vi "Align tilt stages.vi"() -> ()   [LabVIEW 2013]
uses:
  <vilib>/Utility/file.llb/Read From Spreadsheet File (I64).vi
  <vilib>/Utility/file.llb/Write To Spreadsheet File (I64).vi
  <instrlib>/ZaberTSeries/ZaberTSeries.lvlib
panel:
  in  "Load saved position":bool=TRUE
  in  "Save position":bool=TRUE
  in  "Path for saved position":path=path "C:/Users/lab/Documents/GitHub/single-photon-vision/Tools/Calibration/position.txt"
  out "Current position (RV)":i32
  out "Current position (RH)":i32
  in  "Device Number (RH)":u8=4
  in  "Device Number (RV)":u8=3
  out "Current position (LH)":i32
  in  "Device Number (LH)":u8=1
  out "Current position (LV)":i32
  out "error out":errorcluster
  in  "Step Size":i32=1000
  in  "Device Number (LV)":u8=2
  in  "error in (no error)":errorcluster
  in  "VISA resource name":refnum<visa-resource-name>="COM5"
  in  "stop":bool
  # "Press space to update from saved positions."
  # "Press space after STOP to end the VI."
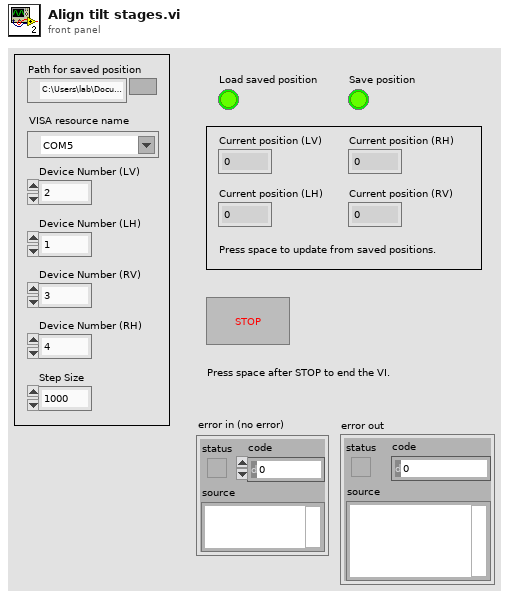
[diagram p1: front panel]
types:
  T1 = enum16{"0", "1", "2", "3", "4", "5", "6", "7", "8", "9", "A", "B", "C", "D", "E", "F", "G", "H", "I", "J", "K", "L", "M", "N", "O", "P", "Q", "R", "S", "T", "U", "V", "W", "X", "Y", "Z", "F1", "F2", "F3", "F4", "F5", "F6", "F7", "F8", "F9", "F10", "F11", "F12", "F13", "F14", "F15", "ADD", "BACK", "BACKSLASH", "CAPITAL", "COMMA", "DECIMAL", "DELETE", "DIVIDE", "DOWN", "END", "EQUALS", "ESCAPE", "GRAVE (`)", "HOME", "INSERT", "LBRACKET", "LCONTROL", "LEFT", "L ALT", "LSHIFT", "LWIN", "MINUS", "MULTIPLY", "NEXT", "NUMLOCK", "NUMPAD_0", "NUMPAD_1", "NUMPAD_2", "NUMPAD_3", "NUMPAD_4", "NUMPAD_5", "NUMPAD_6", "NUMPAD_7", "NUMPAD_8", "NUMPAD_9", "PAUSE", "PERIOD", "PRIOR (PG UP)", "RBRACKET", "RCONTROL", "RETURN", "RIGHT", "R ALT", "RSHIFT", "RWIN", "SCROLL", "SEMICOLON", "SLASH", "SPACE", "SUBTRACT", "TAB", "UP", "ENTER (num pad)", "' (quote)"}
  T2 = cluster{"Response Count":i32, "Command":u8, "Response Count":i32, "Response Count":i32}
  T3 = typedef "ZaberTSeries.lvlib/Response.ctl" = cluster{"Device Number":u8, "Command":u8, "Data":i32}
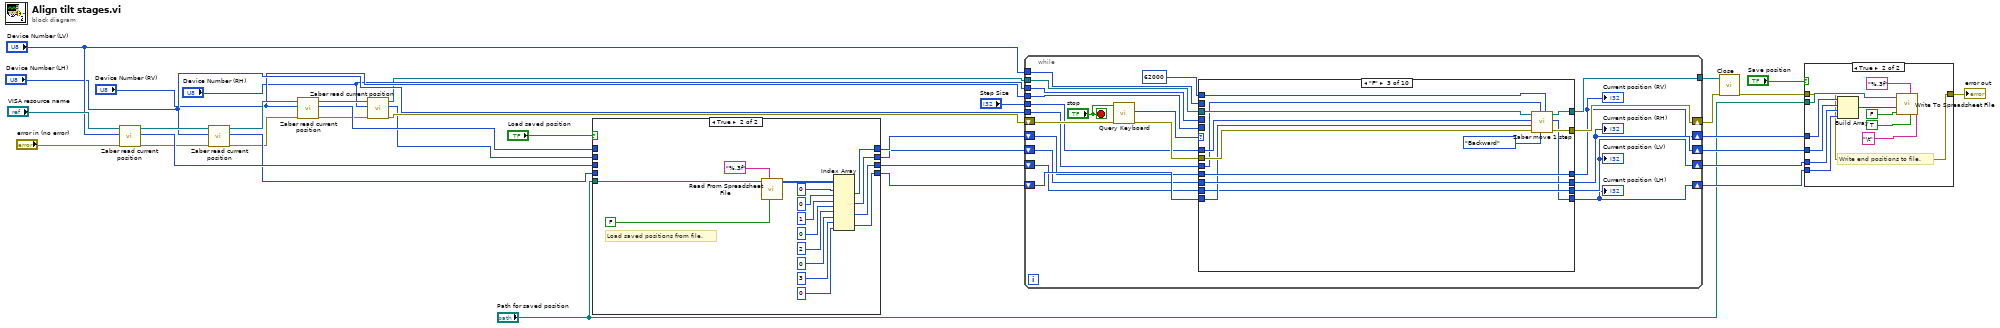
[diagram p0: block diagram]
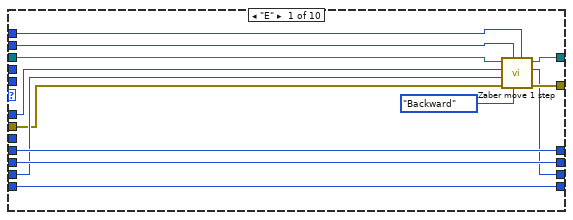
[diagram p4: hidden frame]
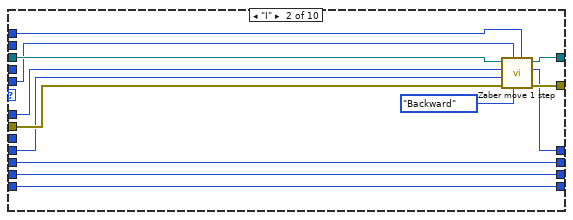
[diagram p5: hidden frame]
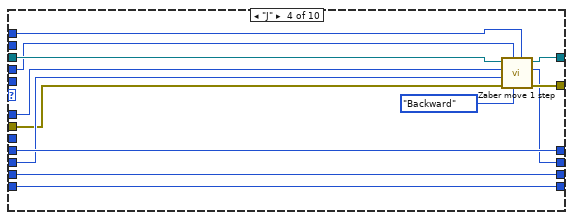
[diagram p6: hidden frame]
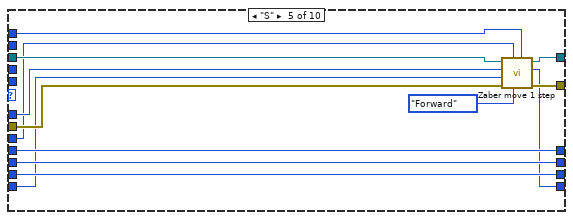
[diagram p7: hidden frame]
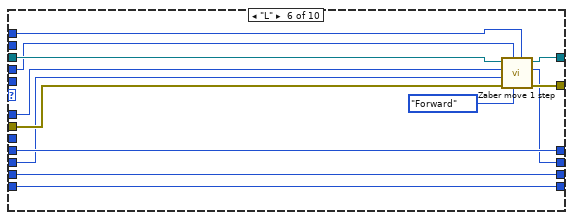
[diagram p8: hidden frame]
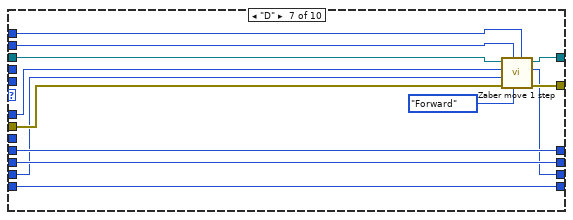
[diagram p9: hidden frame]
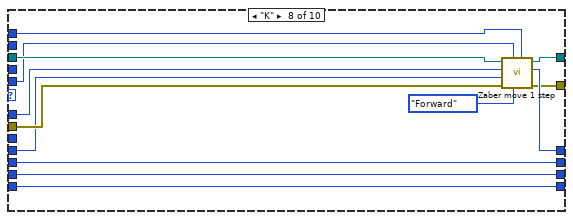
[diagram p10: hidden frame]
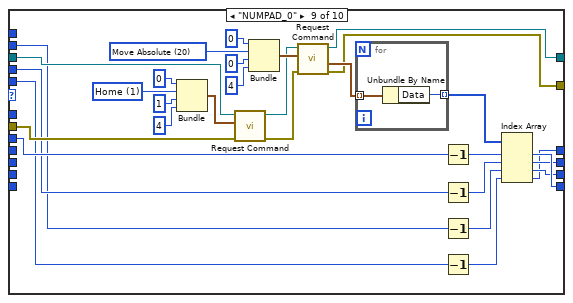
[diagram p11: hidden frame]
diagram:
  n1 = call "Zaber read current position.vi"("error in (no error)"="error in (no error)", "Device Number (LV)"="Device Number (LV)", "VISA Refnum in"="VISA resource name") -> ("error out"=w14:errorcluster, "Current position (LV)"=w18:i32, "VISA Refnum out"=w13:refnum<visa-resource-name>)  [unwired: 6 in]
  n2 = call "Zaber read current position.vi"("error in (no error)"=w14, "Device Number (LV)"="Device Number (LH)", "VISA Refnum in"=w13) -> ("error out"=w10:errorcluster, "Current position (LV)"=w11:i32, "VISA Refnum out"=w9:refnum<visa-resource-name>)  [unwired: 6 in]
  n3 = call "Zaber read current position.vi"("error in (no error)"=w10, "Device Number (LV)"="Device Number (RV)", "VISA Refnum in"=w9) -> ("error out"=w6:errorcluster, "Current position (LV)"=w7:i32, "VISA Refnum out"=w5:refnum<visa-resource-name>)  [unwired: 6 in]
  n4 = call "Zaber read current position.vi"("error in (no error)"=w6, "Device Number (LV)"="Device Number (RH)", "VISA Refnum in"=w5) -> ("error out"=w3:errorcluster, "Current position (LV)"=w2:i32, "VISA Refnum out"=w1:refnum<visa-resource-name>)  [unwired: 6 in]
  n5 = case shown="True" "Load saved position" {
    tunnel: "Path for saved position" -> [_ w54]
    tunnel: w7 -> [w38 _]
    tunnel: [w38 w43] -> w19
    tunnel: w18 -> [w37 _]
    tunnel: [w37 w41] -> w17
    tunnel: [w36 w40] -> w16
    tunnel: w11 -> [w36 _]
    tunnel: [w35 w42] -> w15
    tunnel: w2 -> [w35 _]
    frame False {
    }
    frame True {
      # "Load saved positions from file."
      n6 = call-poly <vilib>:"Read From Spreadsheet File.vi"("transpose (no:F)"=FALSE, "format (%d)"="%.3f" ("format (%.3f)"), "file path (dialog if empty)"=w54) -> ("all rows"=w39:i64[][])  [unwired: 4 in, 4 out]
      n7 = Index Array(array=w39, index (row) #1=0 ("index"), index (col) #1=0 ("disabled index (col)"), index (row) #2=1 ("index"), index (col) #2=0 ("disabled index (col)"), index (row) #3=2 ("index"), index (col) #3=0 ("disabled index (col)"), index (row) #4=3 ("index"), index (col) #4=0 ("disabled index (col)")) -> (element #1=w43:i64, element #2=w42:i64, element #3=w41:i64, element #4=w40:i64)
    }
  }
  n8 = while {
    shift-right: [w73] -> w32
    shift-left: w3 -> [w75]
    tunnel: "Step Size" -> [w71]
    tunnel: "Device Number (LV)" -> [w70]
    tunnel: w1 -> [w69]
    tunnel: [w68] -> w29
    shift-right: [w67] -> w26
    shift-left: w17 -> [w63]
    shift-right: [w65] -> w25
    shift-left: w16 -> [w64]
    tunnel: "Device Number (LH)" -> [w62]
    tunnel: "Device Number (RH)" -> [w59]
    tunnel: "Device Number (RV)" -> [w61]
    shift-right: [w58] -> w27
    shift-left: w15 -> [w57]
    shift-right: [w56] -> w28
    shift-left: w19 -> [w60]
    stop <- "stop" stop-if-true
    n9 = call "Query Keyboard.vi"("error in (no error)"=w75, "Stop?"="stop") -> ("error out"=w74:errorcluster, "element"=w72:T1)  [unwired: 8 in]
    n10 = case shown="\"F\"" w72 {
      tunnel: w74 -> [w80 w98 w111 w121 w137 w149 w162 w176 w205 w217]
      tunnel: [w79 w101 w106 w120 w136 w143 w155 w168 w182 w217] -> w73
      tunnel: w69 -> [w84 w100 w103 w126 w133 w146 w159 w175 w206 w216]
      tunnel: w71 -> [w82 w97 w109 w122 w130 w147 w160 w172 _ _]
      tunnel: w70 -> [w85 _ _ _ _ _ w157 _ w194 _]
      tunnel: [w78 w99 w107 w119 w134 w142 w156 w167 w180 w216] -> w68
      tunnel: [w77 w91 w105 w116 w138 w151 w154 w177 w193 w215] -> w67
      tunnel: w63 -> [w81 w91 w105 w116 w138 w151 w161 w177 _ w215]
      tunnel: 62000 ("Data") -> [w83 w90 w110 w123 w132 w150 w158 w174 _ _]
      tunnel: [w88 w96 w104 w115 w135 w152 w166 w179 w201 w214] -> w65
      tunnel: w64 -> [w88 w96 w108 w115 w131 w152 w166 w179 _ w214]
      tunnel: w62 -> [_ _ w102 _ w129 _ _ _ w200 _]
      tunnel: w61 -> [_ w93 _ _ _ _ _ w173 w191 _]
      tunnel: w60 -> [w86 w92 w113 w127 w139 w153 w164 w170 _ w212]
      tunnel: w59 -> [_ _ _ w124 _ w145 _ _ w197 _]
      tunnel: [w87 w95 w114 w118 w140 w141 w165 w178 w196 w213] -> w58
      tunnel: w57 -> [w87 w95 w114 w125 w140 w148 w165 w178 _ w213]
      tunnel: [w86 w94 w113 w127 w139 w153 w164 w171 w190 w212] -> w56
      frame "E" {
        n11 = call "Zaber move 1 step.vi"("Maximum"=w83, "Direction"=enum16{"Forward", "Backward"}."Backward", "Device Number"=w85, "error in (no error)"=w80, "Current position in"=w81, "Step Size"=w82, "VISA Refnum in"=w84) -> ("error out"=w79:errorcluster, "Current position out"=w77:i64, "VISA Refnum out"=w78:refnum<visa-resource-name>)  [unwired: 2 in]
      }
      frame "I" {
        n12 = call "Zaber move 1 step.vi"("Maximum"=w90, "Direction"=enum16{"Forward", "Backward"}."Backward", "Device Number"=w93, "error in (no error)"=w98, "Current position in"=w92, "Step Size"=w97, "VISA Refnum in"=w100) -> ("error out"=w101:errorcluster, "Current position out"=w94:i64, "VISA Refnum out"=w99:refnum<visa-resource-name>)  [unwired: 2 in]
      }
      frame "F" {
        n13 = call "Zaber move 1 step.vi"("Maximum"=w110, "Direction"=enum16{"Forward", "Backward"}."Backward", "Device Number"=w102, "error in (no error)"=w111, "Current position in"=w108, "Step Size"=w109, "VISA Refnum in"=w103) -> ("error out"=w106:errorcluster, "Current position out"=w104:i64, "VISA Refnum out"=w107:refnum<visa-resource-name>)  [unwired: 2 in]
      }
      frame "J" {
        n14 = call "Zaber move 1 step.vi"("Maximum"=w123, "Direction"=enum16{"Forward", "Backward"}."Backward", "Device Number"=w124, "error in (no error)"=w121, "Current position in"=w125, "Step Size"=w122, "VISA Refnum in"=w126) -> ("error out"=w120:errorcluster, "Current position out"=w118:i64, "VISA Refnum out"=w119:refnum<visa-resource-name>)  [unwired: 2 in]
      }
      frame "S" {
        n15 = call "Zaber move 1 step.vi"("Maximum"=w132, "Direction"=enum16{"Forward", "Backward"}."Forward", "Device Number"=w129, "error in (no error)"=w137, "Current position in"=w131, "Step Size"=w130, "VISA Refnum in"=w133) -> ("error out"=w136:errorcluster, "Current position out"=w135:i64, "VISA Refnum out"=w134:refnum<visa-resource-name>)  [unwired: 2 in]
      }
      frame "L" {
        n16 = call "Zaber move 1 step.vi"("Maximum"=w150, "Direction"=enum16{"Forward", "Backward"}."Forward", "Device Number"=w145, "error in (no error)"=w149, "Current position in"=w148, "Step Size"=w147, "VISA Refnum in"=w146) -> ("error out"=w143:errorcluster, "Current position out"=w141:i64, "VISA Refnum out"=w142:refnum<visa-resource-name>)  [unwired: 2 in]
      }
      frame "D" {
        n17 = call "Zaber move 1 step.vi"("Maximum"=w158, "Direction"=enum16{"Forward", "Backward"}."Forward", "Device Number"=w157, "error in (no error)"=w162, "Current position in"=w161, "Step Size"=w160, "VISA Refnum in"=w159) -> ("error out"=w155:errorcluster, "Current position out"=w154:i64, "VISA Refnum out"=w156:refnum<visa-resource-name>)  [unwired: 2 in]
      }
      frame "K" {
        n18 = call "Zaber move 1 step.vi"("Maximum"=w174, "Direction"=enum16{"Forward", "Backward"}."Forward", "Device Number"=w173, "error in (no error)"=w176, "Current position in"=w170, "Step Size"=w172, "VISA Refnum in"=w175) -> ("error out"=w168:errorcluster, "Current position out"=w171:i64, "VISA Refnum out"=w167:refnum<visa-resource-name>)  [unwired: 2 in]
      }
      frame "NUMPAD_0" {
        w187 = u8 20 items=["Echo"=55, "Home"=1, "Move Absolute"=20, "Move Relative"=21, "Move at Constant Speed"=22, "Renumber"=2, "Restore Settings"=36, "Stop"=23] ("Command")
        w207 = u8 1 items=["Echo"=55, "Home"=1, "Move Absolute"=20, "Move Relative"=21, "Move at Constant Speed"=22, "Renumber"=2, "Restore Settings"=36, "Stop"=23] ("Command")
        n19 = Bundle("Response Count"=0, "Command"=w207, "Response Count"=1, "Response Count"=4) -> (w209:T2)  [unwired: 1 in]
        n20 = call <instrlib>:"Request Command.vi"("error in (no error)"=w205, "Request"=w209, "VISA resource name"=w206) -> ("error out"=w183:errorcluster, "VISA resource name out"=w181:refnum<visa-resource-name>)  [unwired: 5 in, 2 out]
        n21 = Bundle("Response Count"=0, "Command"=w187, "Response Count"=0, "Response Count"=4) -> (w189:T2)  [unwired: 1 in]
        n22 = call <instrlib>:"Request Command.vi"("error in (no error)"=w183, "Request"=w189, "VISA resource name"=w181) -> ("error out"=w182:errorcluster, "Responses out"=w184:T3[], "VISA resource name out"=w180:refnum<visa-resource-name>)  [unwired: 5 in, 1 out]
        n23 = for {
          tunnel: w184 -> [w211] mode=indexing
          tunnel: [w210] -> w202 mode=indexing
          n24 = Unbundle By Name(w211) -> ("Data"=w210:i32)
        }
        n25 = Decrement(x=w200) -> (x-1=w199:u8)
        n26 = Decrement(x=w197) -> (x-1=w198:u8)
        n27 = Decrement(x=w194) -> (x-1=w195:u8)
        n28 = Decrement(x=w191) -> (x-1=w192:u8)
        n29 = Index Array(array=w202, index #1=w199, index #2=w198, index #3=w195, index #4=w192) -> (element #1=w201:i32, element #2=w196:i32, element #3=w193:i32, element #4=w190:i32)
      }
      frame "SPACE", Default {
      }
    }
    "Current position (LV)" <- w67
    "Current position (LH)" <- w65
    "Current position (RH)" <- w58
    "Current position (RV)" <- w56
  }
  n30 = call <instrlib>:"Close.vi"("error in (no error)"=w32, "VISA resource name"=w29) -> ("error out"=w24:errorcluster)  [unwired: 8 in, 1 out]
  n31 = case shown="True" "Save position" {
    tunnel: w28 -> [_ w229]
    tunnel: w27 -> [_ w228]
    tunnel: w26 -> [_ w227]
    tunnel: w25 -> [_ w226]
    tunnel: "Path for saved position" -> [_ w225]
    tunnel: w24 -> [w218 w219]
    tunnel: [w218 w219] -> w23
    frame False {
    }
    frame True {
      # "Write end positions to file."
      n32 = Build Array(w229, w228, w227, w226) -> (w220:i64[])
      n33 = call-poly <vilib>:"Write To Spreadsheet File.vi"("delimiter (\\t)"="\t" ("delimiter (\\t)"), "transpose? (no:F)"=TRUE, "format (%d)"="%.3f" ("format (%.3f)"), "append to file? (new file:F)"=FALSE, "1D data"=w220, "file path (dialog if empty)"=w225) -> ()  [unwired: 2 in, 1 out]
    }
  }
  "error out" <- w23
